vi "Flatten Value.vi"(8 "error in (no error)":errorcluster, 11 "Boolean in":refnum<class "I32 1D.lvclass">) -> (0 "error out":errorcluster, 2 "Value":string, 3 "Boolean out":refnum<class "I32 1D.lvclass">)   [LabVIEW 2019, in "I32 1D.lvclass"]
uses:
  <vilib>/gpm_packages/@cs/data-type-serializer/source/I32 1D/I32 1D.lvclass
  <vilib>/gpm_packages/@cs/data-type-serializer/source/I32 1D/I32 1D.lvclass/I32 1D.ctl
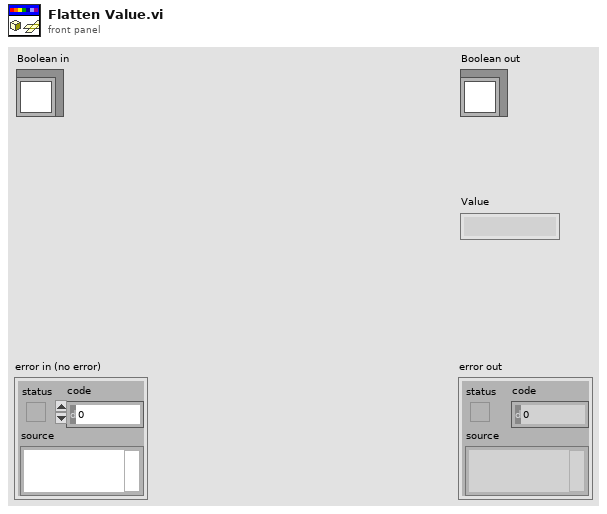
[diagram p1: front panel]
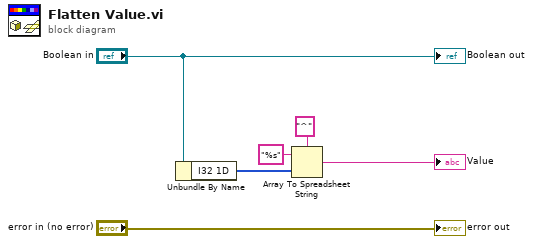
[diagram p0: block diagram]
diagram:
  n1 = Unbundle By Name("Boolean in") -> ("I32 1D"=w4:i32[])
  n2 = Array To Spreadsheet String(delimiter (Tab)="^", array=w4, 3:"%s" ("format string")) -> (spreadsheet string=→"Value":string)
  "error out" <- "error in (no error)"
  "Boolean out" <- "Boolean in"
